vi "Mehrzeilige Texte formatieren.vi"(7 "Zurück formatieren":bool, 11 "string":string caption="String") -> (3 "result string":string caption="Ergebnis-String")   [LabVIEW 2015, in "Sprachverwaltung.lvlib"]
uses:
  Sprachverwaltung.lvlib
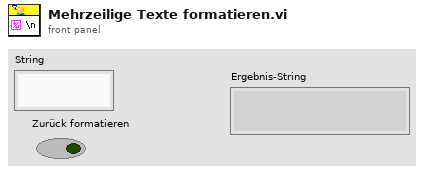
[diagram p1: front panel]
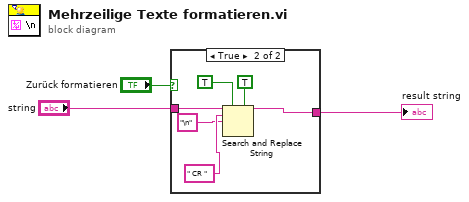
[diagram p0: block diagram]
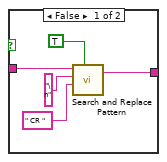
[diagram p2: hidden frame]
diagram:
  n1 = case shown="True" "Zurück formatieren" {
    tunnel: [w8 w13] -> w3
    tunnel: "string" -> [w7 w14]
    frame False {
      n2 = call <vilib>:"Search and Replace Pattern.vi"("string"=w7, "regular expression (\"\")"="\n" ("replace string (\"\")"), "replace string (\"\")"=" CR " ("regular expression (\"\")"), "replace all? (F)"=TRUE) -> ("result string"=w8:string)  [unwired: 1 in, 1 out]
    }
    frame True {
      n3 = Search and Replace String(replace all?=TRUE ("Alle ersetzen? (F)"), multiline?=TRUE ("Mehrzeilig? (F)"), input string=w14, search string=" CR " ("Such-String"), replace string="\n" ("Ersetzungs-String (\"\")")) -> (result string=w13:string)  [unwired: 3 in, 3 out]
    }
  }
  "result string" <- w3
